vi "JTAG Pluto Status.vi"(0 "Address":u16 format="%04x", 11 "error in (no error)":errorcluster) -> (4 "Controller Status":u16 format="%04x", 6 "Charge Active Bit":bool, 8 "Charge Active Status":u16 format="%.0x", 15 "error out":errorcluster)   [LabVIEW 2010]
panel:
  # "ARG1"
  # "ARG2"
  # "ARG3"
  # "ARG4"
  # "ARG5"
  # "ARG6"
  # "ARG7"
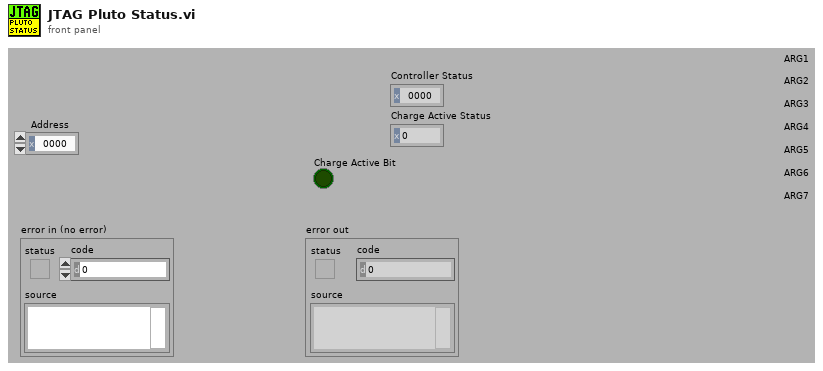
[diagram p1: front panel]
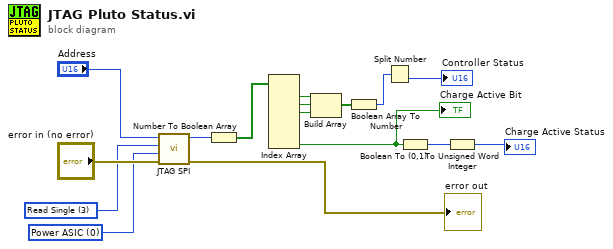
[diagram p0: block diagram]
diagram:
  w12 = u16 0 items=["Power ASIC", "Stim ASIC", "MICS Radio", "FRAM"] ("Target")
  w13 = u16 3 items=["Power UP", "Power DN", "Write Single", "Read Single", "Write Block", "Read Block", "Write Masked", "Test Value"] ("Function")
  n1 = call "JTAG SPI.vi"("error in (no error)"="error in (no error)", "Target"=w12, "Function"=w13, "Address"="Address") -> ("error out"=→"error out":errorcluster, "Read Value"=w11:u8)  [unwired: 4 in, 2 out]
  n2 = Number To Boolean Array(number=w11) -> (Boolean array=w10:bool[])
  n3 = Index Array(array=w10) -> (element #1=w9:bool, element #2=w8:bool, element #3=w7:bool, element #7=w3:bool)  [unwired: 7 in, 3 out]
  "Charge Active Bit" <- w3
  n4 = Build Array(w9, w8, w7) -> (w6:bool[])
  n5 = Boolean Array To Number(Boolean array=w6) -> (number=w5:u32)
  n6 = Split Number(x=w5) -> (lo(x)=→"Controller Status":u16)  [unwired: 1 out]
  n7 = Boolean To (0,1)(Boolean=w3) -> (0, 1=w2:i16)
  n8 = To Unsigned Word Integer(number=w2) -> (unsigned 16bit integer=→"Charge Active Status":u16)
